vi "parseConfigData.vi"(8 "error in (no error)":errorcluster, 11 "results-JSON string":string) -> (0 "error out":errorcluster, 1 "config-text pairs":string[][](array[string]), 2 "config-JSON pairs":string[][](array[string]), 3 "config data":T1)   [LabVIEW 2023, in "Monochromator.lvclass"]
doc: "Converts the JSON config string into a LV cluster"
uses:
  Monochromator.lvclass
  configuration.ctl
  filterWheel.ctl
  grating.ctl
  mirror.ctl
  port.ctl
  41762e30-eae5-4a4c-8725-288ba60ead02.vi
  <vilib>/JDP Science/JSONtext/Next JSON Value.vi
  <vilib>/JDP Science/JSONtext/String Subset.vi
  <vilib>/JDP Science/JSONtext/Parsing/Advance past next JSON Value (inlined COPY).vi
  <vilib>/JDP Science/JSONtext/Parsing/Advance past whitespace.vi
  <vilib>/JDP Science/JSONtext/Parsing/Advance past String.vi
  <vilib>/JDP Science/JSONtext/Parsing/Advance past Number.vi
  <vilib>/JDP Science/JSONtext/Parsing/Advance past Line Ending.vi
  <vilib>/JDP Science/JSONtext/Parsing/Parse Full Path or Item Name.vi
  <vilib>/JDP Science/JSONtext/Parsing/Advance past Array.vi
  <vilib>/JDP Science/JSONtext/Parsing/Advance past Object.vi
  <vilib>/JDP Science/JSONtext/support/Error Cluster From Code.vi
  <vilib>/JDP Science/JSONtext/Offset/Find Item Locations by Path.vi
  <vilib>/JDP Science/JSONtext/JSON text to Variant.vi
  <vilib>/JDP Science/JSONtext/LVClass Serializer/JSONtext LVClass Serializer.lvclass
  <vilib>/JDP Science/JSONtext/JSONtext.lvlib
panel:
  # "Connector Pane"
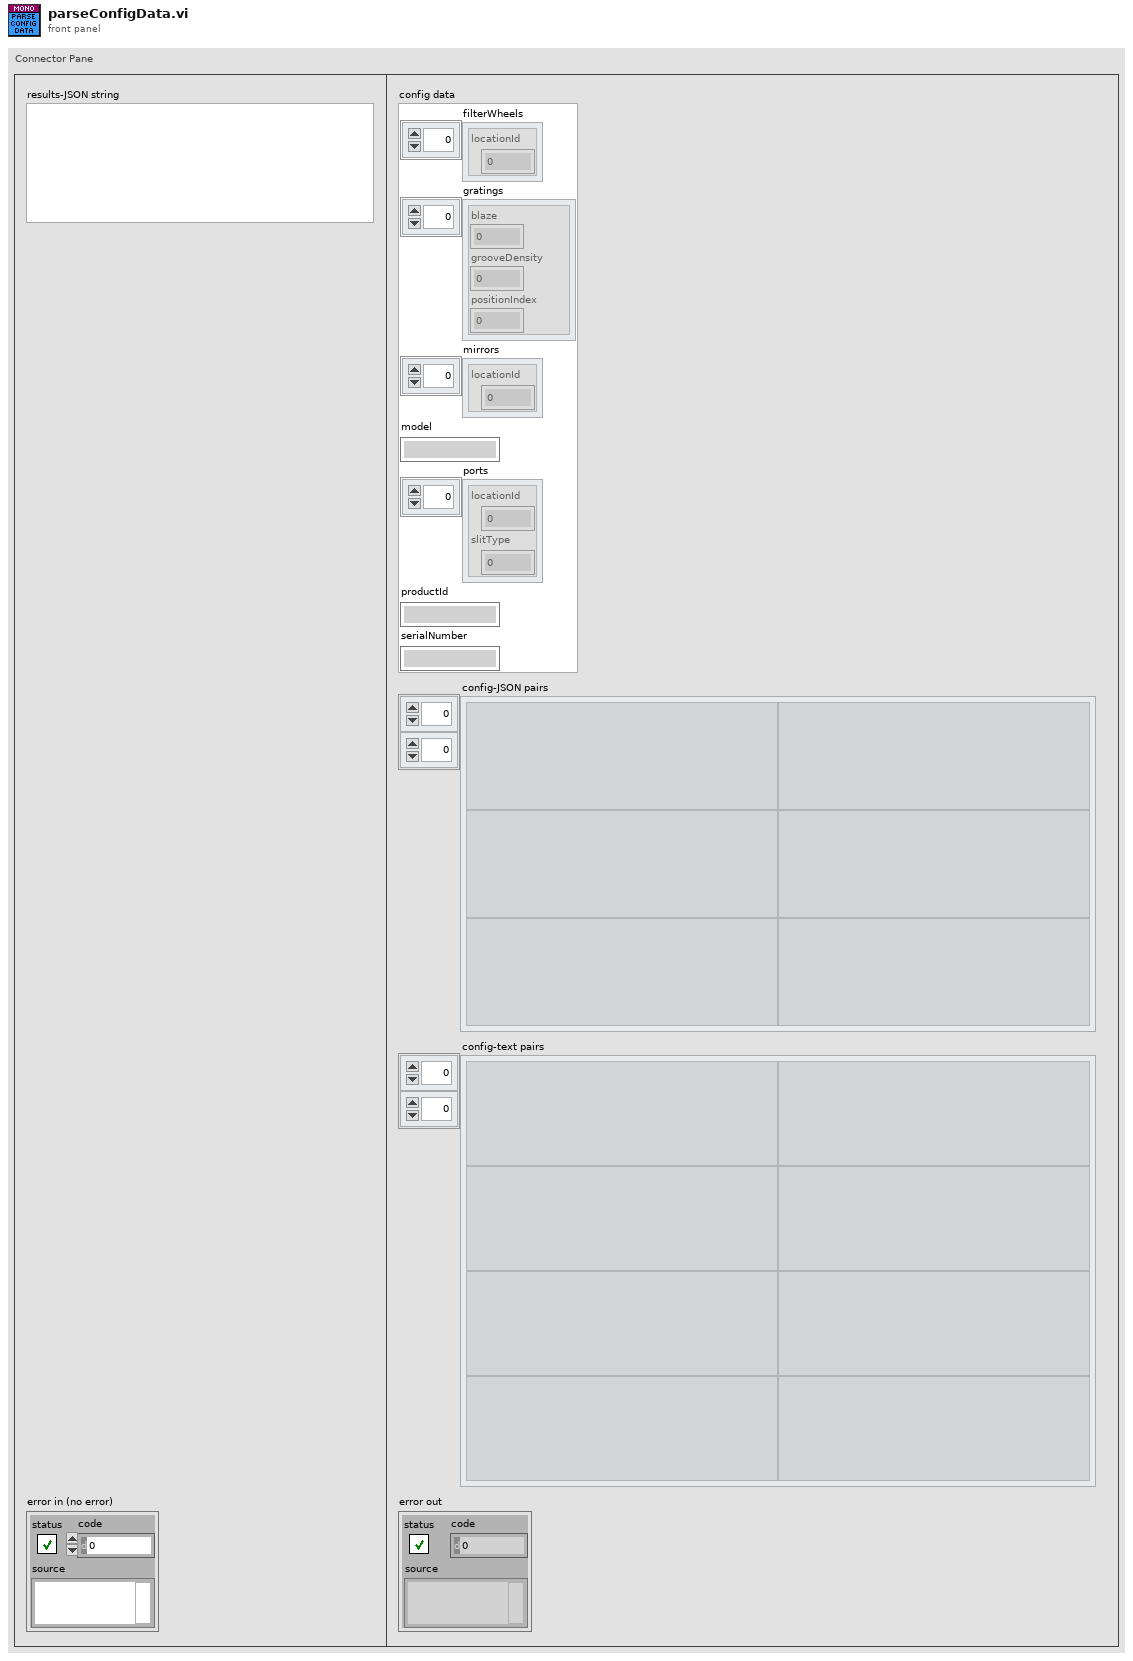
[diagram p1: front panel]
types:
  T1 = typedef "Monochromator.lvclass/configuration.ctl" = cluster{"filterWheels":T2[], "gratings":T3[], "mirrors":T4[], "model":string, "ports":T5[], "productId":string, "serialNumber":string}
  T2 = typedef "Monochromator.lvclass/filterWheel.ctl" = cluster{"locationId":i32}
  T3 = typedef "Monochromator.lvclass/grating.ctl" = cluster{"blaze":i32, "grooveDensity":i32, "positionIndex":i32}
  T4 = typedef "Monochromator.lvclass/mirror.ctl" = cluster{"locationId":i32}
  T5 = typedef "Monochromator.lvclass/port.ctl" = cluster{"locationId":i32, "slitType":i32}
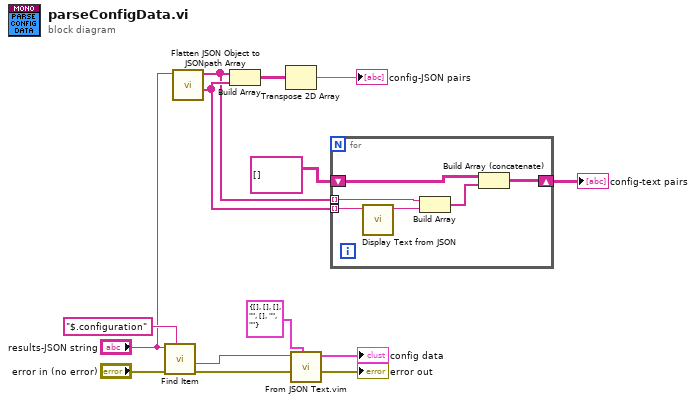
[diagram p0: block diagram]
diagram:
  n1 = call <vilib>:"Find Item.vi"("$Path or Item Name"="$.configuration", "error in (no error)"="error in (no error)", "JSON"="results-JSON string") -> ("error out"=w11:errorcluster, "<JSON>"=w12:string)  [unwired: 5 in, 2 out]
  n2 = call <vilib>:"Flatten JSON Object to JSONpath Array.vi"("JSON"="results-JSON string") -> ("<JSON>"=w5:string[], "$Paths"=w4:string[])  [unwired: 8 in, 1 out]
  n3 = Build Array(w4, w5) -> (w8:string[][])
  n4 = Transpose 2D Array(2D array=w8) -> (transposed array=→"config-JSON pairs":string[][])
  n5 = call "From JSON Text.vim"("Data Type and Default Value"=T1 {"filterWheels"=[], "gratings"=[], "mirrors"=[], "model"="", "ports"=[], "productId"="", "serialNumber"=""} ("configuration"), "error in (no error)"=w11, "JSON"=w12) -> ("error out"=→"error out":errorcluster, "Data out"=→"config data":T1)  [unwired: 7 in]
  n6 = for {
    tunnel: w5 -> [w19] mode=indexing
    tunnel: w4 -> [w18] mode=indexing
    shift-right: [w15] -> w2
    shift-left: string[][] [] -> [w17]
    n7 = call <vilib>:"Display Text from JSON.vi"("Input JSON"=w19) -> ("Display Text"=w20:string)  [unwired: 8 in, 2 out]
    n8 = Build Array(w18, w20) -> (w16:string[])
    n9 = Build Array (concatenate)(w17, w16) -> (w15:string[][])
  }
  "config-text pairs" <- w2
